vi "Mod_OFDM_Frame_bits_to_symbol.vi"(0 "Bits Generated":i8[](array[numeric]), 7 "Parameters per Ofdm Symbol":T1 {"Data Source"."Data Source"."Register Initial State" format="%08x"}, 11 "error in":errorcluster) -> (4 "Complex Mapping":cdb[][](array[numeric]), 8 "Parameters per Ofdm Symbol":T1 {"Data Source"."Data Source"."Register Initial State" format="%08x"}, 15 "error out":errorcluster)   [LabVIEW 2010]
doc: "Complex Mapping of the bits generated are performed based on the modulation scheme selected."
uses:
  Controls(Type_DEf)/Parameters per Ofdm Symbol.ctl
  <vilib>/AddOns/Modulation/Digital/General/MT Generate PSK System Parameters(M).vi
  <vilib>/addons/Modulation/Digital/General/MT Map Bits to PSK Symbols.vi
  <vilib>/AddOns/Modulation/Digital/General/MT Generate QAM System Parameters(M).vi
  <vilib>/addons/Modulation/Digital/General/MT Map Bits to QAM Symbols.vi
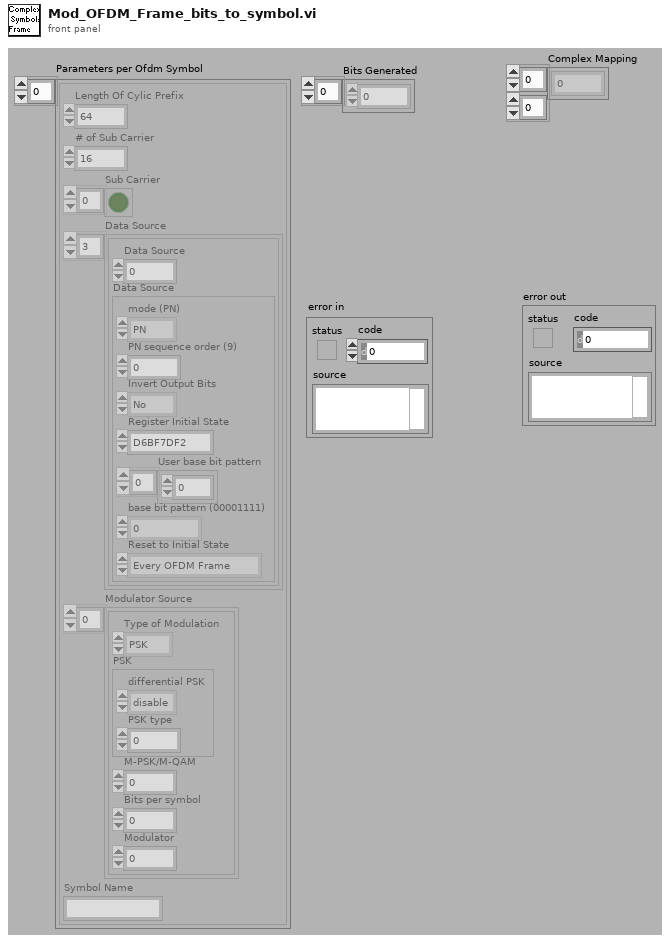
[diagram p1: front panel]
types:
  T1 = typedef "Parameters per Ofdm Symbol.ctl" = cluster{"Length Of Cylic Prefix":i32, "# of Sub Carrier":i32, "Sub Carrier":bool[], "Data Source":cluster{"Data Source":u16, "Data Source":cluster{"mode (PN)":enum16{"PN", "pattern", "user"}, "PN sequence order (9)":i32, "Invert Output Bits":enum16{"No", "Yes"}, "Register Initial State":u32, "User base bit pattern":i8[], "base bit pattern (00001111)":enum16{"0", "1", "01", "0011", "00001111"}, "Reset to Initial State":enum16{"Every OFDM Frame", "Every OFDM Symbol", "Every Sub Carrier"}}}[], "Modulator Source":cluster{"Type of Modulation":enum16{"PSK", "QAM"}, "PSK":cluster{"differential PSK":enum16{"disable", "enable"}, "PSK type":u16}, "M-PSK/M-QAM":i32, "Bits per symbol":i32, "Modulator":u16}[], "Symbol Name":string}[]
  T2 = cluster{"Type of Modulation":enum16{"PSK", "QAM"}, "PSK":cluster{"differential PSK":enum16{"disable", "enable"}, "PSK type":u16}, "M-PSK/M-QAM":i32, "Bits per symbol":i32, "Modulator":u16}[]
  T3 = cluster{"differential PSK":enum16{"disable", "enable"}, "PSK type":u16}
  T4 = cluster{"samples per symbol (16)":i32, "symbol map":cdb[], "differential PSK":enum16{"disable", "enable"}, "PSK type":u16}
  T5 = cluster{"samples per symbol (16)":i32, "symbol map":cdb[]}
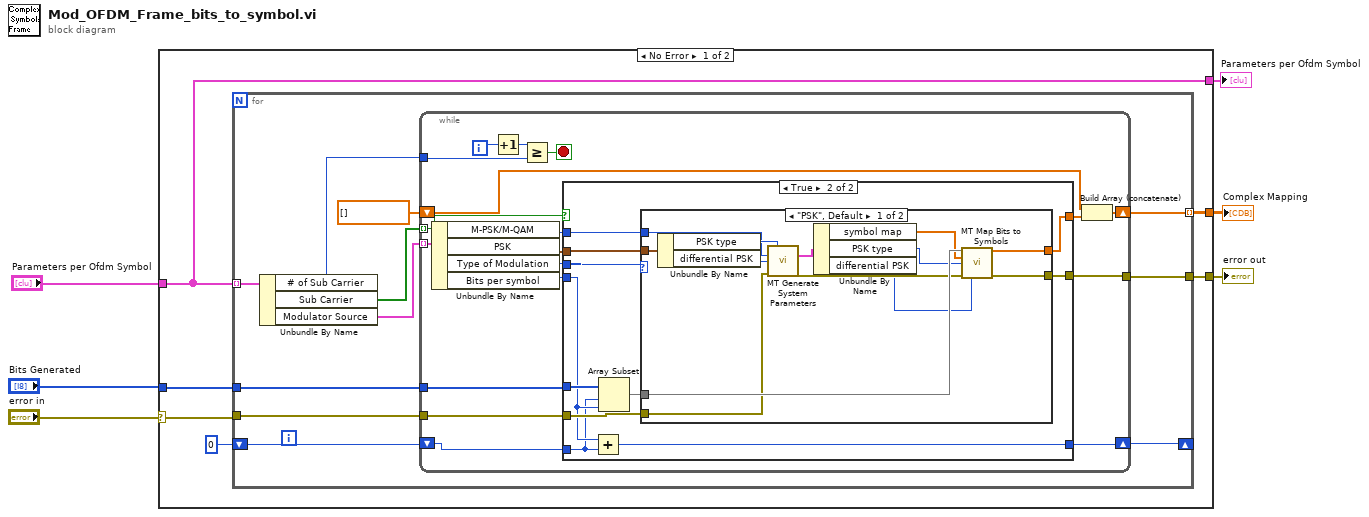
[diagram p0: block diagram]
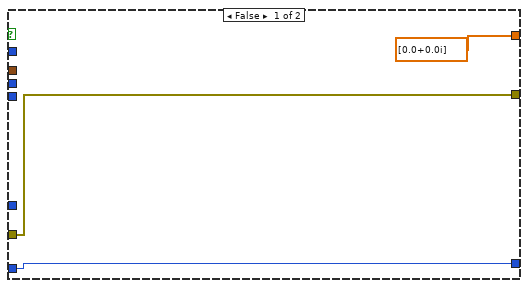
[diagram p2: hidden frame]
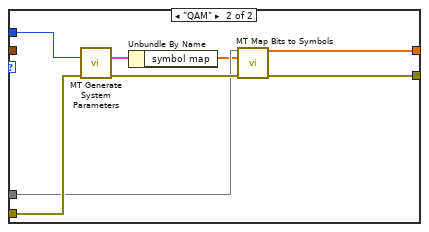
[diagram p3: hidden frame]
diagram:
  n1 = case shown="No Error" "error in" {
    selector: "error in" -> [w10 w77]
    tunnel: [w12 w77] -> w6
    tunnel: [w11 _] -> w5
    tunnel: "Parameters per Ofdm Symbol" -> [w9 _]
    tunnel: [w9 _] -> w2
    tunnel: "Bits Generated" -> [w7 _]
    frame No Error {
      n2 = for {
        tunnel: w10 -> [w22]
        tunnel: [w21] -> w12
        tunnel: [w20] -> w11 mode=indexing
        tunnel: w9 -> [w19] mode=indexing
        shift-right: [w14] -> _
        shift-left: 0 -> [w13]
        tunnel: w7 -> [w15]
        n3 = Unbundle By Name(w19) -> ("# of Sub Carrier"=w18:i32, "Sub Carrier"=w17:bool[], "Modulator Source"=w16:T2)
        n4 = while {
          tunnel: w16 -> [w28] mode=indexing
          tunnel: w17 -> [w38] mode=indexing
          tunnel: w18 -> [w40]
          tunnel: w15 -> [w36]
          tunnel: w22 -> [w34]
          tunnel: [w33] -> w21
          shift-right: [w32] -> w20
          shift-left: cdb[] [] -> [w31]
          shift-right: [w25] -> w14
          shift-left: w13 -> [w24]
          i -> [w30]
          stop <- w39 stop-if-true
          n5 = Unbundle By Name(w28) -> ("M-PSK/M-QAM"=w29:i32, "PSK"=w35:T3, "Type of Modulation"=w37:enum16{"PSK", "QAM"}, "Bits per symbol"=w27:i32)
          n6 = Increment(x=w30) -> (x+1=w41:i32)
          n7 = Greater Or Equal?(x=w41, y=w40) -> (x >= y?=w39:bool)
          n8 = case shown="True" w38 {
            tunnel: w37 -> [_ w48]
            tunnel: w36 -> [_ w54]
            tunnel: w24 -> [w44 w46]
            tunnel: [w44 w55] -> w25
            tunnel: w35 -> [_ w52]
            tunnel: w34 -> [w43 w51]
            tunnel: [w43 w50] -> w33
            tunnel: [cdb[] [0.0+0.0i] ("symbols") w49] -> w26
            tunnel: w29 -> [_ w45]
            tunnel: w27 -> [_ w47]
            frame False {
            }
            frame True {
              n9 = Add(x=w47, y=w46) -> (x+y=w55:i32)
              n10 = Array Subset(array=w54, index=w46, length=w47) -> (w53:i8[])
              n11 = case shown="\"PSK\", Default" w48 {
                tunnel: w53 -> [w67 w73]
                tunnel: w52 -> [w68 _]
                tunnel: [w66 w72] -> w49
                tunnel: [w63 w75] -> w50
                tunnel: w51 -> [w62 w74]
                tunnel: w45 -> [w60 w71]
                frame "PSK", Default {
                  n12 = Unbundle By Name(w68) -> ("PSK type"=w61:u16, "differential PSK"=w65:enum16{"disable", "enable"})
                  n13 = call-poly <vilib>:"MT Generate System Parameters.vi"("PSK type"=w61, "M-PSK (4)"=w60, "differential PSK"=w65, "error in (no error)"=w62) -> ("PSK system parameters"=w59:T4, "error out"=w64:errorcluster)  [unwired: 9 in, 1 out]
                  n14 = Unbundle By Name(w59) -> ("symbol map"=w58:cdb[], "PSK type"=w57:u16, "differential PSK"=w56:enum16{"disable", "enable"})
                  n15 = call-poly <vilib>:"MT Map Bits to Symbols.vi"("input bit stream"=w67, "symbol map"=w58, "PSK type"=w57, "error in (no error)"=w64, "differential PSK"=w56) -> ("symbols"=w66:cdb[], "error out"=w63:errorcluster)  [unwired: 9 in]
                }
                frame "QAM" {
                  n16 = call-poly <vilib>:"MT Generate System Parameters.vi"("M-QAM (16)"=w71, "error in (no error)"=w74) -> ("QAM system parameters"=w70:T5, "error out"=w76:errorcluster)  [unwired: 11 in, 1 out]
                  n17 = Unbundle By Name(w70) -> ("symbol map"=w69:cdb[])
                  n18 = call-poly <vilib>:"MT Map Bits to Symbols.vi"("input bit stream"=w73, "symbol map"=w69, "error in (no error)"=w76) -> ("symbols"=w72:cdb[], "error out"=w75:errorcluster)  [unwired: 11 in]
                }
              }
            }
          }
          n19 = Build Array (concatenate)(w31, w26) -> (w32:cdb[])
        }
      }
    }
    frame Error {
    }
  }
  "error out" <- w6
  "Complex Mapping" <- w5
  "Parameters per Ofdm Symbol" <- w2
